vi "PID_Controller.vi"() -> ()   [LabVIEW 2024]
uses:
  <vilib>/addons/control/pid/pid.llb/PID Advanced (DBL).vi
  <vilib>/addons/control/pid/NI_PID_pid.lvlib
panel:
  out "Gauge":dbl(knob) scale=0.0..100.0 scale format="%#_3g"
  in  "stop":bool
  out "Waveform Chart":T1(graph)
  out "PV (OUTPUT)":dbl(slide) scale=0.0..100.0
  in  "process parameters":T2={"static gain"=2.5, "lag (s)"=2.5, "deadtime (s)"=0.001, "load"=0.0, "deadband"=0.0, "sensor noise"=0.0, "initial PV"=30.0, "plant noise"=0.0} {"plant noise" format="%.2f"; "initial PV" format="%.2f"; "sensor noise" format="%.2f"; "lag (s)" format="%.2f"; "deadtime (s)" format="%.2f"; "deadband" format="%.1f"; "load" format="%.2f"; "static gain" format="%.2f"}
  in  "PID gains":T3={"proportional gain (Kc)"=1.0, "integral time (Ti, min)"=0.01, "derivative time (Td, min)"=0.0} {"derivative time (Td, min)" format="%.3f"; "integral time (Ti, min)" format="%.3f"; "proportional gain (Kc)" format="%.3f"}
  in  "SP(set point)":dbl(slide) scale=0.0..100.0
  in  "auto? (T)":bool=TRUE
  in  "LCV controller":dbl format="%.2f"
  # "PID Controller"
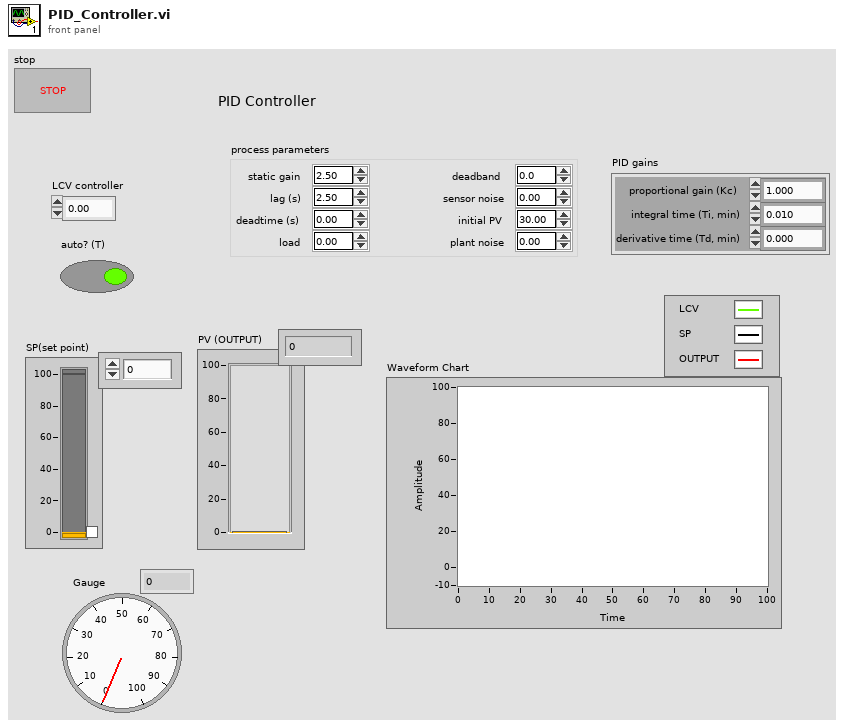
[diagram p1: front panel]
types:
  T1 = cluster{"LCV controller":dbl, "SP(set point)":dbl, "Plant Output":dbl}
  T2 = cluster{"static gain":dbl, "lag (s)":dbl, "deadtime (s)":dbl, "load":dbl, "deadband":dbl, "sensor noise":dbl, "initial PV":dbl, "plant noise":dbl}
  T3 = cluster{"proportional gain (Kc)":dbl, "integral time (Ti, min)":dbl, "derivative time (Td, min)":dbl}
  T4 = cluster{"output":dbl, "SP(set point)":dbl, "Plant Output":dbl}
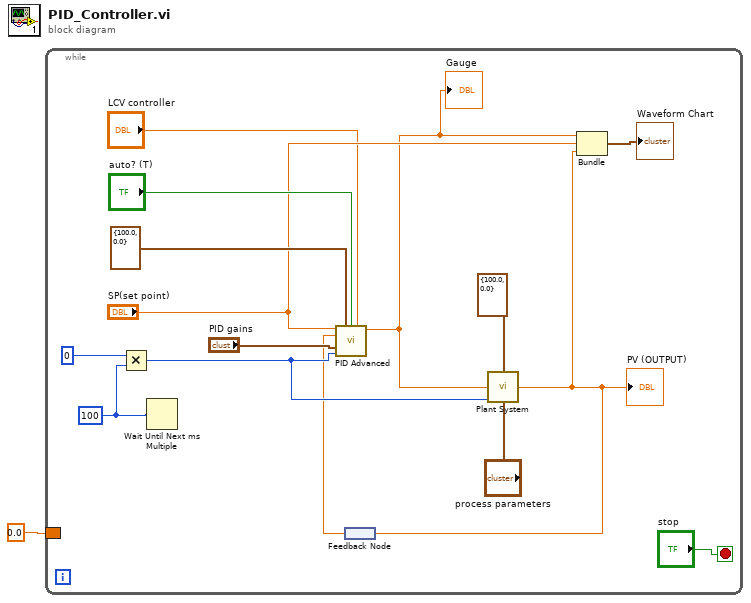
[diagram p0: block diagram]
diagram:
  n1 = while {
    border: 0.0 ("Plant Output") -> [_]
    stop <- "stop" stop-if-true
    w13 = u32 100 ("millisecond multiple")
    n2 = Multiply(x=u32 0, y=w13) -> (x*y=w11:u32)
    n3 = Wait Until Next ms Multiple(millisecond multiple=w13) -> ()  [unwired: 1 out]
    n4 = feedback #1() -> (w8:dbl)
    n5 = call-poly <vilib>:"PID Advanced.vi"("setpoint"="SP(set point)", "output range"=cluster{"output high":dbl, "output low":dbl} {"output high"=100.0, "output low"=0.0}, "auto? (T)"="auto? (T)", "manual control"="LCV controller", "process variable"=w8, "PID gains"="PID gains", "dt (s)"=w11) -> ("output"=w2:dbl)  [unwired: 7 in, 1 out]
    "Gauge" <- w2
    n6 = call "Plant System.vi"("output saturation range"=cluster{"output high":dbl, "output low":dbl} {"output high"=100.0, "output low"=0.0}, "Plant Input"=w2, "dt (s)"=w11, "process parameters"="process parameters") -> ("Plant Output"=w7:dbl)  [unwired: 11 in]
    "PV (OUTPUT)" <- w7
    n7 = feedback-in #1(w7) -> ()
    n8 = Bundle("output"=w2, "SP(set point)"="SP(set point)", "Plant Output"=w7) -> (→"Waveform Chart":T4)  [unwired: 1 in]
  }
